vi "zern2command.vi"(5 "Haso configuration file":path=path "C:/Program Files (x86)/Imagine Optic/Configuration Files/HASO3_first_7364.dat", 6 "idxType":enum16{"Wyant", "ANSI"}(ring), 7 "interaction matrix file":path=path "D:/YD/data/20191206/im.aomi", 8 "error in (no error)":errorcluster, 9 "Zern coef in":sgl[](array[numeric]), 10 "Zern index in":i32[](array[numeric]), 11 "Initial haso file":path=path "D:/SystemAlignment/system_aberration_residual_20191015.has") -> (0 "error out":errorcluster, 1 "Offset Positions":sgl[](array[numeric]), 2 "Zern pupil out":refnum<class "Pupil.lvclass">, 3 "ModalCoef out":refnum<class "ModalCoef.lvclass">)   [LabVIEW 2018]
uses:
  <userlib>/WaveKit.lib/Classes/ModalCoef/ModalCoef.lvclass
  <userlib>/WaveKit.lib/Controls/Pupil.lvclass
  <userlib>/WaveKit.lib/Controls/HasoSlopes.lvclass
  <userlib>/WaveKit.lib/Classes/CorrectionDataManager/CorrectionDataManager.lvclass
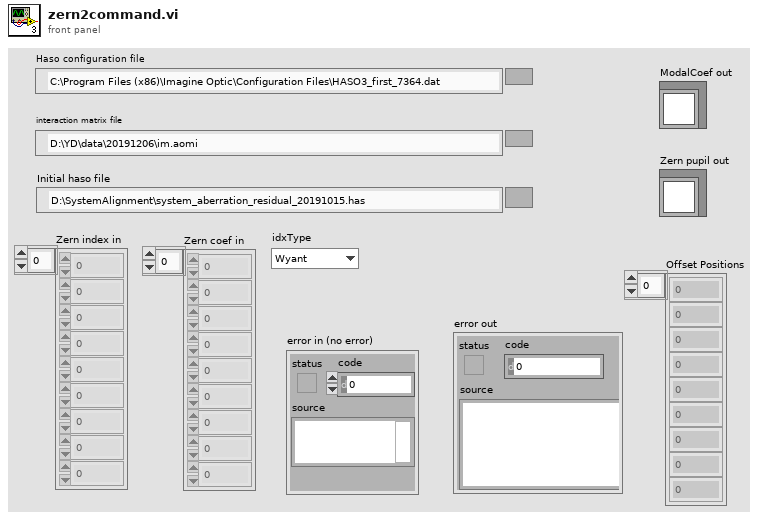
[diagram p1: front panel]
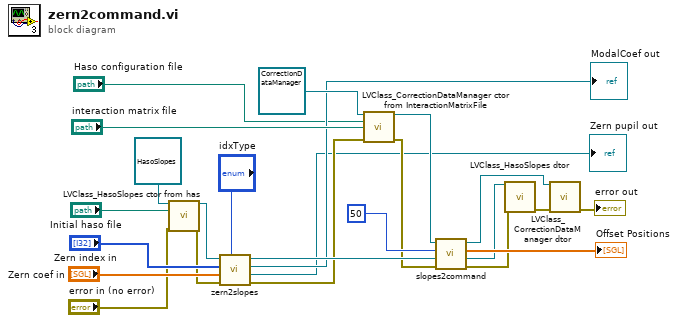
[diagram p0: block diagram]
diagram:
  n1 = call <userlib>:"LVClass_HasoSlopes ctor from has.vi"("HasoSlopes in"=refnum<class "HasoSlopes.lvclass"> refnum, ".has path"="Initial haso file", "error in (no error)"="error in (no error)") -> ("HasoSlopes out"=w17:refnum<class "HasoSlopes.lvclass">, "error out"=w16:errorcluster)  [unwired: 11 in]
  n2 = call "zern2slopes.vi"("idxType"="idxType", "error in (no error)"=w16, "Zern coef in"="Zern coef in", "Zern index in"="Zern index in", "HasoSlopes in"=w17) -> ("error out"=w10:errorcluster, "Zern pupil out"=→"Zern pupil out":refnum<class "Pupil.lvclass">, "ModalCoef out"=→"ModalCoef out":refnum<class "ModalCoef.lvclass">, "HasoSlopes out"=w24:refnum<class "HasoSlopes.lvclass">)  [unwired: 3 in]
  n3 = call <userlib>:"LVClass_CorrectionDataManager ctor from InteractionMatrixFile.vi"("CorrectionDataManager in"=refnum<class "CorrectionDataManager.lvclass"> refnum, "Haso config file path"="Haso configuration file", "Interaction matrix path"="interaction matrix file", "error in (no error)"=w10) -> ("CorrectionDataManager out"=w11:refnum<class "CorrectionDataManager.lvclass">, "error out"=w9:errorcluster)  [unwired: 10 in]
  n4 = call "slopes2command.vi"("error in (no error)"=w9, "HasoSlopes in"=w24, "Number of kept modes"=50, "CorrectionDataManager in"=w11) -> ("error out"=w7:errorcluster, "HasoSlopes out"=w14:refnum<class "HasoSlopes.lvclass">, "Offset Positions"=→"Offset Positions":sgl[], "CorrectionDataManager out"=w8:refnum<class "CorrectionDataManager.lvclass">)  [unwired: 4 in]
  n5 = call <userlib>:"LVClass_HasoSlopes dtor.vi"("HasoSlopes in"=w14, "error in (no error)"=w7) -> ("error out"=w6:errorcluster)  [unwired: 12 in, 1 out]
  n6 = call <userlib>:"LVClass_CorrectionDataManager dtor.vi"("CorrectionDataManager in"=w8, "error in (no error)"=w6) -> ("error out"=→"error out":errorcluster)  [unwired: 12 in, 1 out]
